vi "AMPM Measure.vi"(0 "RFmx Handle In":refnum<k21>, 1 "Selector String":string, 11 "error in (no error)":errorcluster) -> (4 "RFmx Handle Out":refnum<k21>, 6 "AMPM Results":T1 {"AM to PM Residual (deg)" format="%.2f"; "AM to AM Residual (dB)" format="%.2f"; "Mean RMS EVM (%)" format="%.2f"; "1 dB Compression Point (dBm)" format="%.2f"; "Mean Linear Gain (dB)" format="%.2f"}, 15 "error out":errorcluster)   [LabVIEW 2018, in "RFmxSpecAn.lvlib"]
uses:
  RFmxSpecAn.lvlib
  Typedefs/AMPM Results.ctl
  <vilib>/RFmx/SpecAn/mx/RFmxSpecAn.llb/RFmxSpecAn Select Measurement (Single).vi
  <vilib>/RFmx/SpecAn/mx/RFmxSpecAn.llb/RFmxSpecAn AMPM Fetch DUT Characteristics.vi
  <vilib>/RFmx/SpecAn/mx/RFmxSpecAn.llb/RFmxSpecAn AMPM Fetch Curve Fit Residual.vi
  <vilib>/RFmx/SpecAn/mx/RFmxSpecAn.llb/RFmxSpecAn AMPM Fetch AM to AM Trace.vi
  <vilib>/RFmx/SpecAn/mx/RFmxSpecAn.llb/RFmxSpecAn AMPM Fetch AM to PM Trace.vi
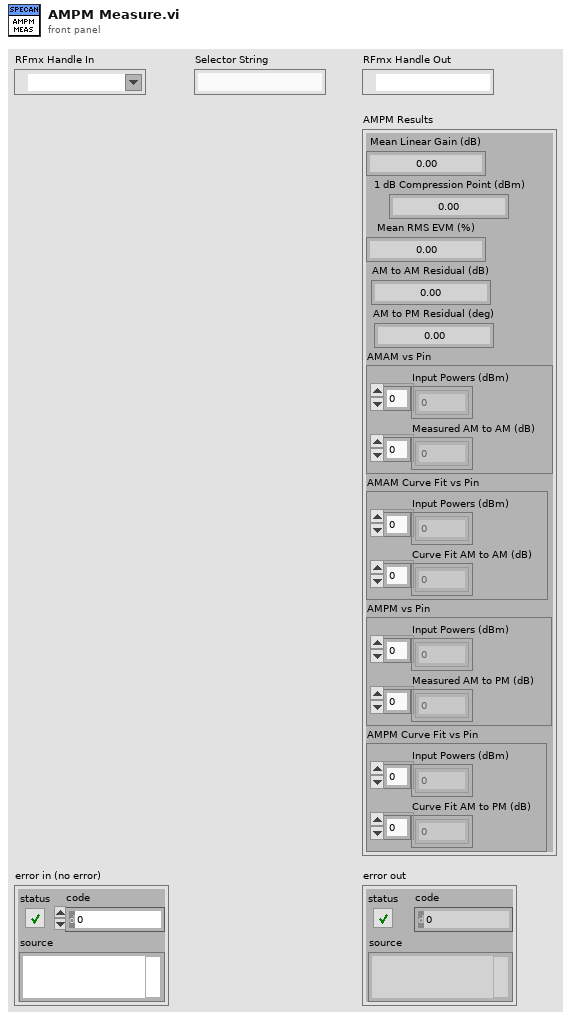
[diagram p1: front panel]
types:
  T1 = typedef "RFmxSpecAn.lvlib/AMPM Results.ctl" = cluster{"Mean Linear Gain (dB)":dbl, "1 dB Compression Point (dBm)":dbl, "Mean RMS EVM (%)":dbl, "AM to AM Residual (dB)":dbl, "AM to PM Residual (deg)":dbl, "AMAM vs Pin":cluster{"Input Powers (dBm)":sgl[], "Measured AM to AM (dB)":sgl[]}, "AMAM Curve Fit vs Pin":cluster{"Input Powers (dBm)":sgl[], "Curve Fit AM to AM (dB)":sgl[]}, "AMPM vs Pin":cluster{"Input Powers (dBm)":sgl[], "Measured AM to PM (dB)":sgl[]}, "AMPM Curve Fit vs Pin":cluster{"Input Powers (dBm)":sgl[], "Curve Fit AM to PM (dB)":sgl[]}}
  T2 = enum16{"ACP", "CCDF", "CHP", "FCnt", "Harmonics", "OBW", "SEM", "Spectrum", "Spur", "TXP", "AMPM", "DPD", "IQ", "IM", "NF", "PhaseNoise"}
  T3 = cluster{"Reference Powers (dBm)":sgl[], "Measured AM to AM (dB)":sgl[]}
  T4 = cluster{"Reference Powers (dBm)":sgl[], "Curve Fit AM to AM (dB)":sgl[]}
  T5 = cluster{"Reference Powers (dBm)":sgl[], "Measured AM to PM (deg)":sgl[]}
  T6 = cluster{"Reference Powers (dBm)":sgl[], "Curve Fit AM to PM (deg)":sgl[]}
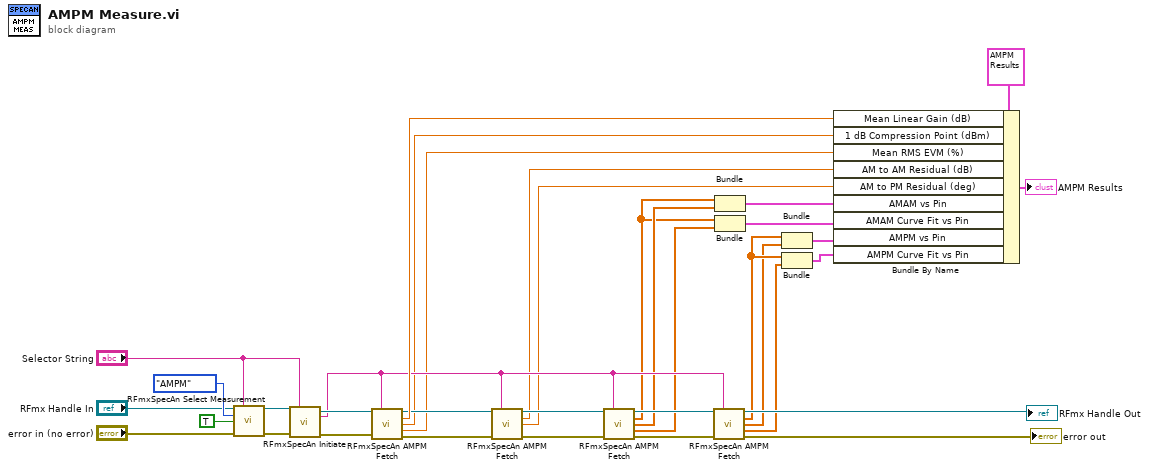
[diagram p0: block diagram]
diagram:
  n1 = call-poly <vilib>:"RFmxSpecAn Select Measurement.vi"("Instrument Handle In"="RFmx Handle In", "Selector String"="Selector String", "Measurement"=T2."AMPM", "Enable All Traces"=TRUE, "error in (no error)"="error in (no error)") -> ("Instrument Handle Out"=w31:refnum<k21>, "error out"=w30:errorcluster)  [unwired: 9 in]
  n2 = call <vilib>:"RFmxSpecAn Initiate.vi"("Instrument Handle In"=w31, "Selector String"="Selector String", "error in (no error)"=w30) -> ("Instrument Handle Out"=w27:refnum<k21>, "Selector String Out"=w15:string, "error out"=w28:errorcluster)  [unwired: 10 in]
  n3 = call-poly <vilib>:"RFmxSpecAn AMPM Fetch.vi"("Instrument Handle In"=w27, "Selector String"=w15, "error in (no error)"=w28) -> ("Instrument Handle Out"=w21:refnum<k21>, "Mean Linear Gain (dB)"=w24:dbl, "1 dB Compression Point (dBm)"=w13:dbl, "Mean RMS EVM (%)"=w12:dbl, "error out"=w26:errorcluster)  [unwired: 8 in]
  n4 = call-poly <vilib>:"RFmxSpecAn AMPM Fetch.vi"("Instrument Handle In"=w21, "Selector String"=w15, "error in (no error)"=w26) -> ("Instrument Handle Out"=w19:refnum<k21>, "AM to AM Residual (dB)"=w11:dbl, "AM to PM Residual (deg)"=w10:dbl, "error out"=w22:errorcluster)  [unwired: 9 in]
  n5 = call-poly <vilib>:"RFmxSpecAn AMPM Fetch.vi"("Instrument Handle In"=w19, "Selector String"=w15, "error in (no error)"=w22) -> ("Instrument Handle Out"=w17:refnum<k21>, "Reference Powers (dBm)"=w7:sgl[], "Measured AM to AM (dB)"=w14:sgl[], "Curve Fit AM to AM (dB)"=w8:sgl[], "error out"=w20:errorcluster)  [unwired: 8 in]
  n6 = call-poly <vilib>:"RFmxSpecAn AMPM Fetch.vi"("Instrument Handle In"=w17, "Selector String"=w15, "error in (no error)"=w20) -> ("Instrument Handle Out"=→"RFmx Handle Out":refnum<k21>, "Reference Powers (dBm)"=w3:sgl[], "Measured AM to PM (deg)"=w2:sgl[], "Curve Fit AM to PM (deg)"=w1:sgl[], "error out"=→"error out":errorcluster)  [unwired: 8 in]
  n7 = Bundle("Reference Powers (dBm)"=w7, "Measured AM to AM (dB)"=w14) -> (w9:T3)  [unwired: 1 in]
  n8 = Bundle("Reference Powers (dBm)"=w7, "Curve Fit AM to AM (dB)"=w8) -> (w6:T4)  [unwired: 1 in]
  n9 = Bundle("Reference Powers (dBm)"=w3, "Measured AM to PM (deg)"=w2) -> (w5:T5)  [unwired: 1 in]
  n10 = Bundle("Reference Powers (dBm)"=w3, "Curve Fit AM to PM (deg)"=w1) -> (w4:T6)  [unwired: 1 in]
  n11 = Bundle By Name(cluster=T1 {"Mean Linear Gain (dB)"=0.0, "1 dB Compression Point (dBm)"=0.0, "Mean RMS EVM (%)"=0.0, "AM to AM Residual (dB)"=0.0, "AM to PM Residual (deg)"=0.0, "AMAM vs Pin"={"Input Powers (dBm)"=[], "Measured AM to AM (dB)"=[]}, "AMAM Curve Fit vs Pin"={"Input Powers (dBm)"=[], "Curve Fit AM to AM (dB)"=[]}, "AMPM vs Pin"={"Input Powers (dBm)"=[], "Measured AM to PM (dB)"=[]}, "AMPM Curve Fit vs Pin"={"Input Powers (dBm)"=[], "Curve Fit AM to PM (dB)"=[]}} ("AMPM Results"), "Mean Linear Gain (dB)"=w24, "1 dB Compression Point (dBm)"=w13, "Mean RMS EVM (%)"=w12, "AM to AM Residual (dB)"=w11, "AM to PM Residual (deg)"=w10, "AMAM vs Pin"=w9, "AMAM Curve Fit vs Pin"=w6, "AMPM vs Pin"=w5, "AMPM Curve Fit vs Pin"=w4) -> (→"AMPM Results":T1)
